vi "nanomsg_ctx_destroy.vi"(3 "error in":errorcluster, 4 "reap? (F)":bool, 5 "context in":refnum<class "nanomsg_context.lvclass">) -> (0 "error out":errorcluster)   [LabVIEW 2014, in "nanomsg.lvlib" / "nanomsg_context.lvclass"]
doc: "Terminates the <b>context</b> fed in. This is a <b>blocking</b> call, and only returns once every socket associated with the context has been terminated."
uses:
  nanomsg_context.lvclass
  nanomsg_context.lvclass/nanomsg_context.ctl
  <vilib>/Utility/error.llb/Error Cluster From Error Code.vi
  nanomsg.lvlib
panel:
  # "NN"
  # "labview"
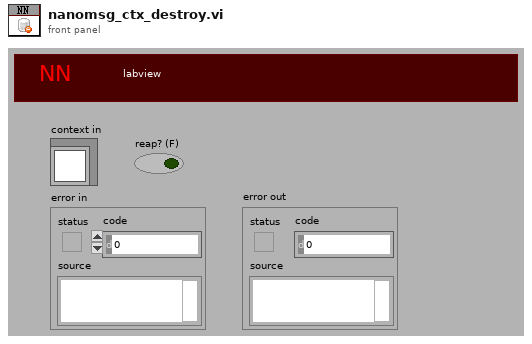
[diagram p1: front panel]
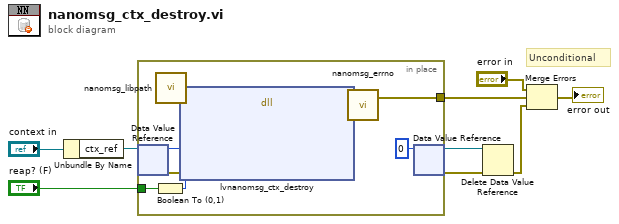
[diagram p0: block diagram]
diagram:
  # "Unconditional"
  n1 = Unbundle By Name("context in") -> ("ctx_ref"=w7:refnum<data-value>)
  n2 = in-place {
    in-place-border: [w18] -> w9
    in-place-border: "reap? (F)" -> [w16]
    n3 = in-place-dvr #1(w7) -> (w17:u64, w12:errorcluster)
    n4 = Boolean To (0,1)(Boolean=w16) -> (0, 1=w15:i16)
    n5 = call "nanomsg_libpath.vi"() -> ("path"=w13:path)
    n6 = dll-call lib="?" fn="lvnanomsg_ctx_destroy" ("zmq_labview.dll:lvzmq_term")(path in=w13, error in=w12, "ctx_obj"=w17, "flags"=w15) -> (error out=w10:errorcluster, "return"=w11:i32)  [unwired: 5 in, 1 out]
    n7 = call "nanomsg_errno.vi"("retval"=w11, "error in"=w10) -> ("error out"=w18:errorcluster)  [unwired: 1 out]
    n8 = in-place-dvr #1(u64 0 ("data value")) -> (w4:refnum<data-value>, w5:errorcluster)
  }
  n9 = Delete Data Value Reference(data value reference=w4, error in=w5) -> (error out=w1:errorcluster)  [unwired: 1 out]
  n10 = Merge Errors("error in", w9, w1) -> (→"error out":errorcluster)
